vi "test jitter.vi"() -> ()   [LabVIEW 2013]
uses:
  <vilib>/gmath/statdist.llb/Normal Random.vi
  <vilib>/gmath/NI_Gmath.lvlib
panel:
  out "jitter estimate":dbl[](graph)
  out "mean period estimate":dbl[](graph)
  in  "period":dbl[unit]=1e-09
  in  "std":dbl[unit]=1e-06
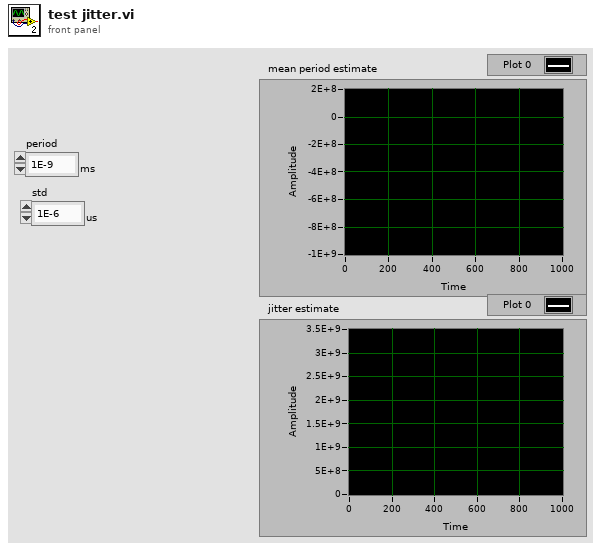
[diagram p1: front panel]
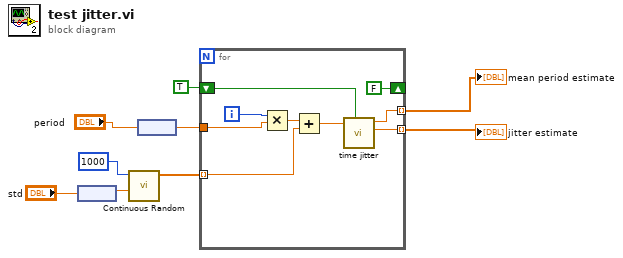
[diagram p0: block diagram]
diagram:
  n1 = node("std") -> (w4:dbl)
  n2 = call-poly <vilib>:"Continuous Random.vi"("std"=w4, "samples"=1000) -> ("normal random data"=w7:dbl[])  [unwired: 8 in, 1 out]
  n3 = node("period") -> (w5:dbl)
  n4 = for {
    tunnel: w7 -> [w16] mode=indexing
    tunnel: w5 -> [w15]
    tunnel: [w13] -> w3 mode=indexing
    tunnel: [w12] -> w2 mode=indexing
    shift-right: [FALSE] -> _
    shift-left: TRUE -> [w11]
    i -> [w18]
    n5 = Multiply(x=w18, y=w15) -> (x*y=w17:dbl)
    n6 = Add(x=w17, y=w16) -> (x+y=w14:dbl)
    n7 = call "time jitter.vi"("reset"=w11, "time (ns)"=w14) -> ("jitter"=w12:dbl, "mean period"=w13:dbl)  [unwired: 8 in]
  }
  "mean period estimate" <- w3
  "jitter estimate" <- w2
